vi "pb_start_programming.vi"(8 "error in (no error)":errorcluster, 10 "Device":T1(ring), 11 "path in":path=path "C:/Program Files/SpinCore/SpinAPI/dll/spinapi.dll") -> (0 "error out":errorcluster, 3 "path out":path)   [LabVIEW 2018]
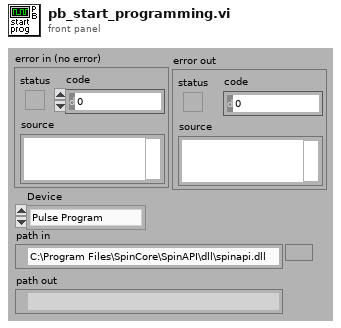
[diagram p1: front panel]
types:
  T1 = enum16{"Pulse Program", "Frequency Registers", "TX Phase Registers", "RX Phase Registers"}
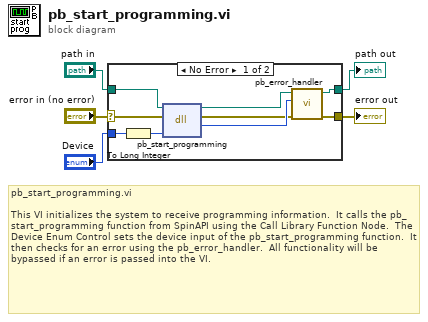
[diagram p0: block diagram]
diagram:
  # "pb_start_programming.vi\n\nThis VI initializes the system to receive programming information.  It calls the pb_start_programming function from SpinAPI using the Call Library Function Node.  The Device Enum Control sets the device input of the pb_start_programming function.  It then checks for an error using the pb_error_handler.  All functionality will be bypassed if an error is passed into the VI."
  n1 = case shown="No Error" "error in (no error)" {
    selector: "error in (no error)" -> [w11 w16]
    tunnel: [w6 w16] -> w5
    tunnel: "Device" -> [w13 _]
    tunnel: "path in" -> [w10 w15]
    tunnel: [w7 w15] -> w1
    frame No Error {
      n2 = To Long Integer(number=w13) -> (32bit integer=w12:i32)
      n3 = dll-call lib="C:/Program Files/SpinCore/SpinAPI/dll/spinapi.dll" fn="pb_start_programming"(path in=w10, error in=w11, "device"=w12) -> (path out=w8:path, error out=w9:errorcluster, "return type"=w14:i32)  [unwired: 2 in]
      n4 = call "pb_error_handler.vi"("error in (no error)"=w9, "return code"=w14, "path in"=w8) -> ("error out"=w6:errorcluster, "path out"=w7:path)  [unwired: 7 out]
    }
    frame Error {
    }
  }
  "error out" <- w5
  "path out" <- w1
